vi "norm! (SubVI).vi"(0 "start coord":cluster{"x":dbl, "y":dbl}={"x"=40.0, "y"=40.0}, 1 "goal coord":cluster{"x":dbl, "y":dbl}={"x"=40.0, "y"=40.0}, 6 "seed":i32=-1, 7 "samples":i32=-1, 8 "upper limit":cluster{"x":dbl, "y":dbl}={"x"=40.0, "y"=40.0}, 9 "std":dbl=1.0, 10 "mean":dbl, 11 "reset":bool=TRUE) -> (3 "Array":cluster{"x":dbl, "y":dbl}[](array[cluster]))   [LabVIEW 2011]
uses:
  <vilib>/gmath/statdist.llb/Normal Random.vi
  <vilib>/gmath/NI_Gmath.lvlib
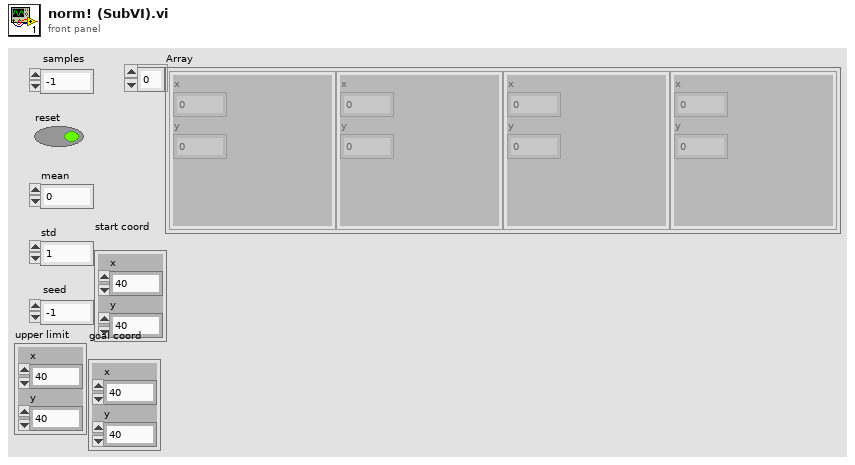
[diagram p1: front panel]
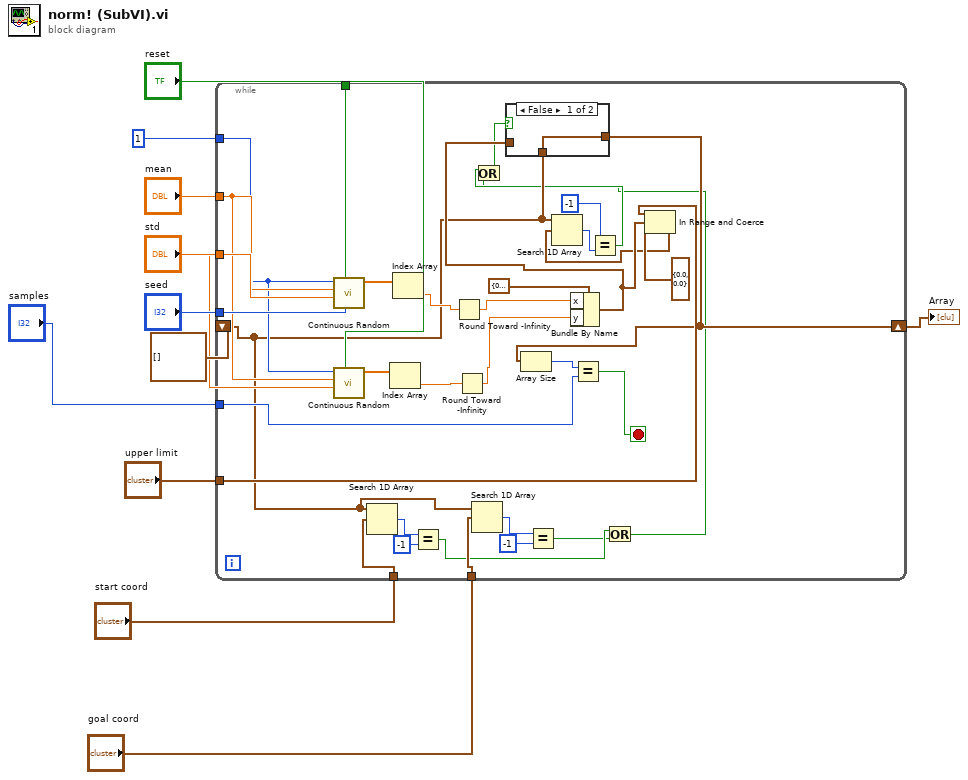
[diagram p0: block diagram]
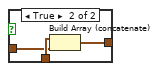
[diagram p2: hidden frame]
diagram:
  n1 = while {
    tunnel: "seed" -> [w45]
    tunnel: "std" -> [w44]
    tunnel: "mean" -> [w43]
    tunnel: 1 ("samples") -> [w42]
    tunnel: "reset" -> [w41]
    shift-right: [w24] -> w11
    shift-left: cluster{"x":dbl, "y":dbl}[] [] -> [w23]
    tunnel: "samples" -> [w34]
    tunnel: "upper limit" -> [w25]
    tunnel: "start coord" -> [w22]
    tunnel: "goal coord" -> [w21]
    stop <- w33 stop-if-true
    n2 = call-poly <vilib>:"Continuous Random.vi"("seed"=w45, "reset"=w41, "std"=w44, "mean"=w43, "samples"=w42) -> ("normal random data"=w39:dbl[])  [unwired: 5 in, 1 out]
    n3 = call-poly <vilib>:"Continuous Random.vi"("reset"=w41, "std"=w44, "mean"=w43, "samples"=w42) -> ("normal random data"=w38:dbl[])  [unwired: 6 in, 1 out]
    n4 = Search 1D Array(1D array=w23, element=w22) -> (index of element=w20:i32)  [unwired: 1 in]
    n5 = Index Array(array=w38) -> (element=w31:dbl)  [unwired: 1 in]
    n6 = Index Array(array=w39) -> (element=w32:dbl)  [unwired: 1 in]
    n7 = Equal?(x=w20, y=-1) -> (x = y?=w16:bool)
    n8 = Round Toward -Infinity(1:w32) -> (0:w29:dbl)
    n9 = Round Toward -Infinity(1:w31) -> (0:w30:dbl)
    n10 = Search 1D Array(1D array=w23, element=w21) -> (index of element=w18:i32)  [unwired: 1 in]
    n11 = Equal?(x=w18, y=-1) -> (x = y?=w15:bool)
    n12 = Bundle By Name(cluster=cluster{"x":dbl, "y":dbl} {"x"=0.0, "y"=0.0} ("input cluster"), "x"=w29, "y"=w30) -> (w28:cluster{"x":dbl, "y":dbl})
    n13 = Or(x=w16, y=w15) -> (x .or. y?=w13:bool)
    n14 = In Range and Coerce(upper limit=w25, x=w28, lower limit=cluster{"x":dbl, "y":dbl} {"x"=0.0, "y"=0.0}) -> (coerced(x)=w26:cluster{"x":dbl, "y":dbl})  [unwired: 1 out]
    n15 = Search 1D Array(1D array=w23, element=w26) -> (index of element=w37:i32)  [unwired: 1 in]
    n16 = Equal?(x=-1 ("y"), y=w37) -> (x = y?=w14:bool)
    n17 = Or(x=w14, y=w13) -> (x .or. y?=w12:bool)
    n18 = case shown="False" w12 {
      tunnel: w28 -> [_ w48]
      tunnel: w23 -> [w46 w49]
      tunnel: [w46 w47] -> w24
      frame False {
      }
      frame True {
        n19 = Build Array (concatenate)(w49, w48) -> (w47:cluster{"x":dbl, "y":dbl}[])
      }
    }
    n20 = Array Size(array=w24) -> (size(s)=w35:i32)
    n21 = Equal?(x=w35, y=w34) -> (x = y?=w33:bool)
  }
  "Array" <- w11
